vi "Insight_Select_Laser.vi"(8 "error in (no error)":errorcluster) -> (0 "error out":errorcluster, 3 "IP address":string="192.168.1.100")   [LabVIEW 2014]
doc: "Insight Photonic Solutions\nCopyright 2014\n\nThis VI enables the user to discover the laser on a network, or select the laser at a particular IP address.\n\nver 1.0 - Original Release"
panel:
  in  "Lasers Found":bool
  in  "Laser Search":enum32{"Searching", "Available Lasers"}(tab)
  out "Search Indicator":cluster{u8, u8}(slide)={0, 49} scale=0.0..100.0
  in  "refresh":bool
  in  "IP address":string="192.168.1.100"
  in  "select":bool
  in  "Available Lasers":i32(listbox)
  in  "cancel":bool
  # "Searching for lasers..."
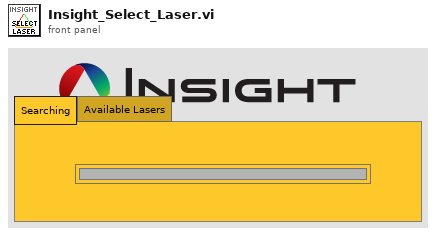
[diagram p1: front panel]
types:
  T1 = enum32{"Invalid", "Default", "Floating", "Floating/Auto-Hide", "Modal"}
  T2 = enum8{"Enabled", "Disabled", "Disabled and Grayed Out"}
  T3 = cluster{"IP Address":string, "Serial Number":string}[]
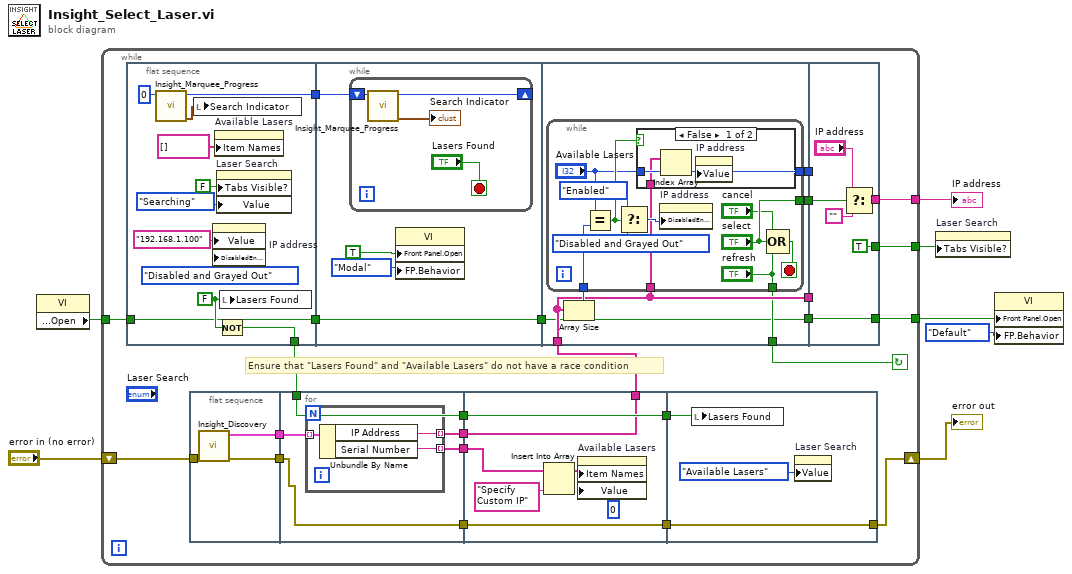
[diagram p0: block diagram]
diagram:
  n1 = property class="VI"() -> ("Front Panel.Open"=w2:bool)  [unwired: 2 in, 2 out]
  n2 = while {
    tunnel: [w18] -> w7
    tunnel: [w17] -> w6
    tunnel: [w15] -> w4
    shift-right: [w14] -> w3
    shift-left: "error in (no error)" -> [w16]
    tunnel: w2 -> [w11]
    stop <- w13 continue-if-true
    # "Ensure that \"Lasers Found\" and \"Available Lasers\" do not have a race condition"
    n3 = flat-sequence {
      tunnel: [w41] -> w20
      tunnel: [w34] -> w12
      tunnel: w11 -> [w32]
      tunnel: [w32] -> w10
      tunnel: w12 -> [w46]
      tunnel: w10 -> [w44]
      tunnel: [w44] -> w9
      tunnel: [w56] -> w23
      tunnel: w19 -> [w54]
      tunnel: [w54] -> w22
      tunnel: [w53] -> w21
      tunnel: [w52] -> w13
      tunnel: w9 -> [w51]
      tunnel: [w51] -> w8
      tunnel: w23 -> [_]
      tunnel: w22 -> [_]
      tunnel: [w75] -> w18
      tunnel: [w71] -> w17
      tunnel: [TRUE ("Tabs Visible?")] -> w15
      tunnel: w21 -> [w73]
      tunnel: w8 -> [w71]
      frame #0 {
        w42 = FALSE ("Lasers Found")
        n4 = call "Insight_Marquee_Progress.vi"("x"=u8 0) -> ("Progress Indicator"=w33:cluster{u8, u8}, "x (out)"=w34:u8)  [unwired: 9 in]
        n5 = local write "Search Indicator"(w33) -> ()
        n6 = property on="IP address" class="Str"("Value"="192.168.1.100" ("Custom IP address"), "DisabledEnum"=T2."Disabled and Grayed Out" ("Disabled")) -> ()  [unwired: 2 in, 2 out]
        n7 = property on="Available Lasers" class="LstBox (strict)"("Item Names"=string[] []) -> ()  [unwired: 2 in, 2 out]
        n8 = property on="Laser Search" class="TabCtl (strict)"("Tabs Visible?"=FALSE, "Value"=enum32{"Searching", "Available Lasers"}."Searching" ("Laser Search")) -> ()  [unwired: 2 in, 2 out]
        n9 = Not(x=w42) -> (.not. x?=w41:bool)
        n10 = local write "Lasers Found"(w42) -> ()
      }
      frame #1 {
        n11 = while {
          shift-right: [w48] -> _
          shift-left: w46 -> [w49]
          stop <- "Lasers Found" stop-if-true
          n12 = call "Insight_Marquee_Progress.vi"("x"=w49) -> ("Progress Indicator"=→"Search Indicator":cluster{u8, u8}, "x (out)"=w48:u8)  [unwired: 9 in]
        }
        n13 = property class="VI"("Front Panel.Open"=TRUE ("Front Panel Window:Open"), "FP.Behavior"=T1."Modal" ("Front Panel Window:Behavior")) -> ()  [unwired: 2 in, 2 out]
      }
      frame #2 {
        n14 = Array Size(array=w54) -> (size(s)=w55:i32)
        n15 = while {
          tunnel: w55 -> [w67]
          tunnel: ["Available Lasers"] -> w56
          tunnel: w54 -> [w61]
          tunnel: ["select"] -> w53
          tunnel: ["refresh"] -> w52
          stop <- w60 stop-if-true
          n16 = Equal?(x="Available Lasers", y=w67) -> (x = y?=w63:bool)
          n17 = Select(t=T2."Enabled" ("Disabled"), s=w63, f=T2."Disabled and Grayed Out" ("Disabled")) -> (s? t:f=w66:T2)
          n18 = case shown="False" w63 {
            tunnel: "Available Lasers" -> [w70 _]
            tunnel: w61 -> [w69 _]
            frame False {
              n19 = Index Array(array=w69, index=w70) -> (element=w68:string)
              n20 = property on="IP address" class="Str"("Value"=w68) -> ()  [unwired: 2 in, 2 out]
            }
            frame True {
            }
          }
          n21 = property on="IP address" class="Str"("DisabledEnum"=w66) -> ()  [unwired: 2 in, 2 out]
          n22 = Compound Arithmetic op=OR("cancel", "select", "refresh") -> (w60:bool)
        }
      }
      frame #3 {
        n23 = Select(t="IP address", s=w73, f="") -> (s? t:f=w75:string)
      }
    }
    n24 = flat-sequence {
      tunnel: [w79] -> w31
      tunnel: [w78] -> w30
      tunnel: w16 -> [w77]
      tunnel: [w84] -> w29
      tunnel: w20 -> [w84]
      tunnel: w31 -> [w83]
      tunnel: [w82] -> w28
      tunnel: [w81] -> w27
      tunnel: [w80] -> w26
      tunnel: w30 -> [w80]
      tunnel: w29 -> [w92]
      tunnel: w28 -> [w89]
      tunnel: [w92] -> w25
      tunnel: [w89] -> w19
      tunnel: w27 -> [w90]
      tunnel: [w88] -> w24
      tunnel: w26 -> [w88]
      tunnel: w25 -> [w96]
      tunnel: [w95] -> w14
      tunnel: w24 -> [w95]
      frame #0 {
        n25 = call "Insight_Discovery.vi"("error in (no error)"=w77) -> ("error out"=w78:errorcluster, "Available Lasers"=w79:T3)  [unwired: 9 in]
      }
      frame #1 {
        n26 = for {
          tunnel: w83 -> [w87] mode=indexing
          tunnel: [w86] -> w82 mode=indexing
          tunnel: [w85] -> w81 mode=indexing
          n27 = Unbundle By Name(w87) -> ("IP Address"=w86:string, "Serial Number"=w85:string)
        }
      }
      frame #2 {
        n28 = Insert Into Array(array=w90, new element="Specify Custom IP" ("new element/subarray")) -> (w91:string[])  [unwired: 1 in]
        n29 = property on="Available Lasers" class="LstBox (strict)"("Item Names"=w91, "Value"=0 ("Available Lasers")) -> ()  [unwired: 2 in, 2 out]
      }
      frame #3 {
        n30 = local write "Lasers Found"(w96) -> ()
        n31 = property on="Laser Search" class="TabCtl (strict)"("Value"=enum32{"Searching", "Available Lasers"}."Available Lasers" ("Laser Search")) -> ()  [unwired: 2 in, 2 out]
      }
    }
  }
  "IP address" <- w7
  "error out" <- w3
  n32 = property on="Laser Search" class="TabCtl (strict)"("Tabs Visible?"=w4) -> ()  [unwired: 2 in, 2 out]
  n33 = property class="VI"("Front Panel.Open"=w6, "FP.Behavior"=T1."Default" ("Front Panel Window:Behavior")) -> ()  [unwired: 2 in, 2 out]
